vi "Begin.vi"(11 "Image Size":T1=enum."160x120") -> (0 "error out":errorcluster)   [LabVIEW 2012]
doc: "Called before other user functions, this VI is expected to open initial I/O refnums, load in file data, and do all program initialization. Notice that the <B>error out</B> terminal is simply used for data flow. Wiring it to other structures or subVIs ensures that this VI runs first."
uses:
  <vilib>/Rock Robotics/WPI/Camera/WPI_CameraImageSize.ctl
  <vilib>/Rock Robotics/WPI/DriverStation/WPI_DriverStationRobotMode2.ctl
  <vilib>/Rock Robotics/WPI/Camera/WPI_CameraWhite Balance Values.ctl
  <vilib>/Rock Robotics/WPI/Camera/WPI_CameraExposure Values.ctl
  <vilib>/Rock Robotics/WPI/Camera/WPI_CameraFrameRate.ctl
  Robot Global Data.vi
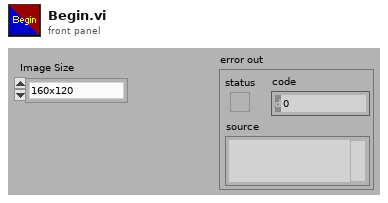
[diagram p1: front panel]
types:
  T1 = typedef "WPI_CameraImageSize.ctl" = enum16{"640x480", "320x240", "160x120"}
  T2 = typedef "WPI_DriverStationRobotMode2.ctl" = enum16{"Autonomous Disabled", "Autonomous Enabled", "Teleop Disabled", "Teleop Enabled", "Timeout", "Finish", "Test Disabled", "Test Enabled"}
  T3 = typedef "WPI_CameraFrameRate.ctl" = u32
  T4 = typedef "WPI_CameraExposure Values.ctl" = enum16{"Auto", "Flicker-free 50 Hz", "Flicker-free 60 Hz", "Hold current"}
  T5 = typedef "WPI_CameraWhite Balance Values.ctl" = enum16{"Auto", "Fixed indoor", "Fixed outdoor 1", "Fixed outdoor 2", "Fixed fluorescent 1", "Fixed fluorescent 2", "Hold current"}
  T6 = typedef "WPI_CameraDevRef.ctl" = cluster{"Camera Address":string, "CameraStatus":errorcluster, "Acquire Image Notifier":refnum<notifier>}
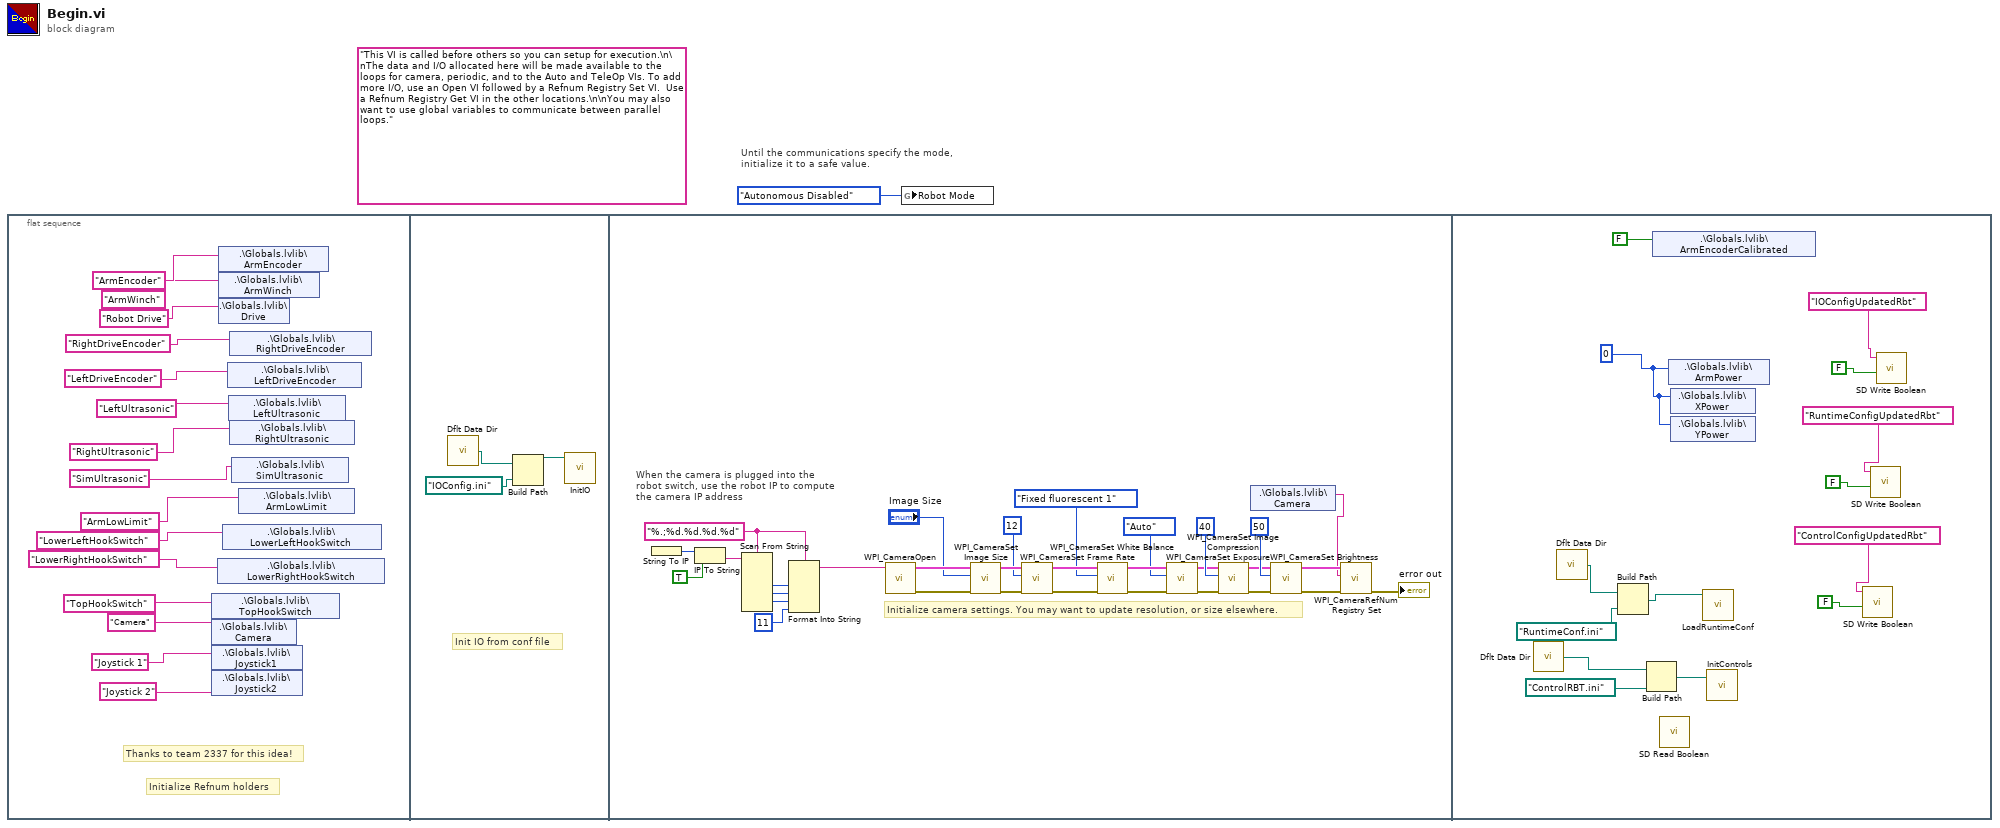
[diagram p0: block diagram]
diagram:
  (unwired) "This VI is called before others so you can setup for execution.\n\nThe data and I/O allocated here will be made available to the loops for camera, periodic, and to the Auto and TeleOp VIs. To add more I/O, use an Open VI followed by a Refnum Registry Set VI.  Use a Refnum Registry Get VI in the other locations.\n\nYou may also want to use global variables to communicate between parallel loops."
  # "Until the communications specify the mode,\ninitialize it to a safe value."
  n1 = flat-sequence {
    frame #0 {
      # "Thanks to team 2337 for this idea!"
      # "Initialize Refnum holders"
      n2 = shared-variable ".\\Globals.lvlib\\TopHookSwitch"("TopHookSwitch") -> ()  [unwired: 1 in, 1 out]
      n3 = shared-variable ".\\Globals.lvlib\\Camera"("Camera") -> ()  [unwired: 1 in, 1 out]
      n4 = shared-variable ".\\Globals.lvlib\\Joystick1"("Joystick 1") -> ()  [unwired: 1 in, 1 out]
      n5 = shared-variable ".\\Globals.lvlib\\Joystick2"("Joystick 2") -> ()  [unwired: 1 in, 1 out]
      n6 = shared-variable ".\\Globals.lvlib\\LowerRightHookSwitch"("LowerRightHookSwitch") -> ()  [unwired: 1 in, 1 out]
      n7 = shared-variable ".\\Globals.lvlib\\ArmEncoder"("ArmEncoder") -> ()  [unwired: 1 in, 1 out]
      n8 = shared-variable ".\\Globals.lvlib\\ArmWinch"("ArmWinch") -> ()  [unwired: 1 in, 1 out]
      n9 = shared-variable ".\\Globals.lvlib\\Drive"("Robot Drive") -> ()  [unwired: 1 in, 1 out]
      n10 = shared-variable ".\\Globals.lvlib\\LowerLeftHookSwitch"("LowerLeftHookSwitch") -> ()  [unwired: 1 in, 1 out]
      n11 = shared-variable ".\\Globals.lvlib\\LeftDriveEncoder"("LeftDriveEncoder") -> ()  [unwired: 1 in, 1 out]
      n12 = shared-variable ".\\Globals.lvlib\\LeftUltrasonic"("LeftUltrasonic") -> ()  [unwired: 1 in, 1 out]
      n13 = shared-variable ".\\Globals.lvlib\\RightDriveEncoder"("RightDriveEncoder") -> ()  [unwired: 1 in, 1 out]
      n14 = shared-variable ".\\Globals.lvlib\\RightUltrasonic"("RightUltrasonic") -> ()  [unwired: 1 in, 1 out]
      n15 = shared-variable ".\\Globals.lvlib\\SimUltrasonic"("SimUltrasonic") -> ()  [unwired: 1 in, 1 out]
      n16 = shared-variable ".\\Globals.lvlib\\ArmLowLimit"("ArmLowLimit") -> ()  [unwired: 1 in, 1 out]
    }
    frame #1 {
      # "Init IO from conf file"
      n17 = call <vilib>:"Dflt Data Dir.vi"() -> ("App:Default Data Directory"=w17:path)
      n18 = Build Path(base path=w17, name or relative path=path "IOConfig.ini") -> (appended path=w19:path)
      n19 = call "InitIO.vi"("Path"=w19) -> ()  [unwired: 11 in]
    }
    frame #2 {
      w23 = "%.;%d.%d.%d.%d" ("format string")
      # "When the camera is plugged into the\nrobot switch, use the robot IP to compute\nthe camera IP address"
      # "Initialize camera settings. You may want to update resolution, or size elsewhere."
      n20 = String To IP() -> (0:w30:u32)  [unwired: 1 in]
      n21 = IP To String(1:TRUE ("dot notation? (F)"), 2:w30) -> (0:w28:string)
      n22 = Scan From String(format string=w23, input string=w28) -> (output 1=w27:i32, output 2=w26:i32, output 3=w25:i32)  [unwired: 7 in, 3 out]
      n23 = Format Into String(format string=w23, w27, w26, w25, 11 ("Compression")) -> (resulting string=w22:string)  [unwired: 2 in, 1 out]
      n24 = call <vilib>:"WPI_CameraOpen.vi"("Camera Address"=w22) -> ("error out"=w42:errorcluster, "CameraDevRef"=w43:T6)  [unwired: 2 in, 7 out]
      n25 = call <vilib>:"WPI_CameraSet Image Size.vi"("error in (no error)"=w42, "Image Size"="Image Size", "CameraDevRef"=w43) -> ("error out"=w41:errorcluster, "CameraDevRef Out"=w44:T6)  [unwired: 7 out]
      n26 = call <vilib>:"WPI_CameraSet Frame Rate.vi"("error in (no error)"=w41, "Frame Rate (fps)"=T3 12, "CameraDevRef"=w44) -> ("error out"=w40:errorcluster, "CameraDevRef Out"=w46:T6)  [unwired: 7 out]
      n27 = call <vilib>:"WPI_CameraSet White Balance.vi"("error in (no error)"=w40, "White Balance"=WPI_CameraWhite_Balance_Values."Fixed fluorescent 1", "CameraDevRef"=w46) -> ("error out"=w39:errorcluster, "CameraDevRef Out"=w45:T6)  [unwired: 7 out]
      n28 = call <vilib>:"WPI_CameraSet Exposure.vi"("error in (no error)"=w39, "Exposure"=WPI_CameraExposure_Values."Auto", "CameraDevRef"=w45) -> ("error out"=w38:errorcluster, "CameraDevRef Out"=w48:T6)  [unwired: 7 out]
      n29 = call <vilib>:"WPI_CameraSet Image Compression.vi"("error in (no error)"=w38, "Compression"=40, "CameraDevRef"=w48) -> ("error out"=w37:errorcluster, "CameraDevRef Out"=w47:T6)  [unwired: 7 out]
      n30 = shared-variable ".\\Globals.lvlib\\Camera"() -> (w20:string)  [unwired: 1 in, 1 out]
      n31 = call <vilib>:"WPI_CameraSet Brightness.vi"("error in (no error)"=w37, "Brightness"=50, "CameraDevRef"=w47) -> ("error out"=w35:errorcluster, "CameraDevRef Out"=w36:T6)  [unwired: 7 out]
      n32 = call <vilib>:"WPI_CameraRefNum Registry Set.vi"("error in (no error)"=w35, "refnum name"=w20, "CameraDevRef"=w36) -> ("error out"=→"error out":errorcluster)  [unwired: 8 out]
    }
    frame #3 {
      w63 = 0
      n33 = call <vilib>:"Dflt Data Dir.vi"() -> ("App:Default Data Directory"=w53:path)
      n34 = call <vilib>:"Dflt Data Dir.vi"() -> ("App:Default Data Directory"=w60:path)
      n35 = Build Path(base path=w60, name or relative path=path "RuntimeConf.ini") -> (appended path=w58:path)
      n36 = Build Path(base path=w53, name or relative path=path "ControlRBT.ini") -> (appended path=w52:path)
      n37 = shared-variable ".\\Globals.lvlib\\ArmEncoderCalibrated"(FALSE) -> ()  [unwired: 1 in, 1 out]
      n38 = call <vilib>:"SD Read Boolean.vi"() -> ()  [unwired: 9 in, 3 out]
      n39 = shared-variable ".\\Globals.lvlib\\ArmPower"(w63) -> ()  [unwired: 1 in, 1 out]
      n40 = shared-variable ".\\Globals.lvlib\\XPower"(w63) -> ()  [unwired: 1 in, 1 out]
      n41 = shared-variable ".\\Globals.lvlib\\YPower"(w63) -> ()  [unwired: 1 in, 1 out]
      n42 = call "LoadRuntimeConf.vi"("Path"=w58) -> ()  [unwired: 11 in]
      n43 = call "InitControls.vi"("Config"=w52) -> ()  [unwired: 11 in]
      n44 = call <vilib>:"SD Write Boolean.vi"("Boolean"=FALSE, "Name"="ControlConfigUpdatedRbt") -> ()  [unwired: 8 in, 2 out]
      n45 = call <vilib>:"SD Write Boolean.vi"("Boolean"=FALSE, "Name"="RuntimeConfigUpdatedRbt") -> ()  [unwired: 8 in, 2 out]
      n46 = call <vilib>:"SD Write Boolean.vi"("Boolean"=FALSE, "Name"="IOConfigUpdatedRbt") -> ()  [unwired: 8 in, 2 out]
    }
  }
  n47 = global write "Robot Global Data.vi" "Robot Mode"(WPI_DriverStationRobotMode2."Autonomous Disabled" ("Robot Mode")) -> ()
